vi "Actor Core Contents.vi"(8 "error in":errorcluster, 11 "Actor in":refnum<class "Actor.lvclass">) -> (0 "error out":errorcluster, 3 "Actor out":refnum<class "Actor.lvclass">)   [LabVIEW 2026, in "Lumberjack.lvlib" / "LogManager.lvclass"]
doc: "<p>(<strong>Filename</strong>: <span class=\"dnl\">Actor Framework.lvlib:Actor.lvclass:Actor Core.vi</span>)</p>\n<p>Receives messages to the actor, reacts to them, and initiates any error handling that may shut the actor down.</p>\n<p>Descendant classes may override this VI to append parallel tasks for the actor to complete while it handles messages. Overrides use the <a href=\"nihelplauncher://docs/csh?context=lvcore_glang_udclass\">Call Parent Class Method</a> node.</p>"
uses:
  LogManager.lvclass
  LogManager.lvclass/LogManager.ctl
  Appenders/Appender.lvclass/Appender.lvclass
  <vilib>/ActorFramework/Actor/Actor.lvclass
  C:/Program Files (x86)/National Instruments/LabVIEW 2026/vi.lib/ActorFramework/Actor/Actor.lvclass
  C:/Users/dallis/OneDrive - Velico Medical/Documents/Personal/LabVIEW Coding Projects/Lumberjack/src/Core/LogManager/LogManager.lvclass/LogManager.lvclass
  Layouts/CSVLayout.lvclass/CSVLayout.lvclass
  C:/Users/dallis/OneDrive - Velico Medical/Documents/Personal/LabVIEW Coding Projects/Lumberjack/src/Core/Layouts/Layout.lvclass/Layout.lvclass
  C:/Users/dallis/OneDrive - Velico Medical/Documents/Personal/LabVIEW Coding Projects/Lumberjack/src/Core/Layouts/CSVLayout.lvclass/CSVLayout.lvclass
  Appenders/FileAppender.lvclass/FileAppender.lvclass
  C:/Users/dallis/OneDrive - Velico Medical/Documents/Personal/LabVIEW Coding Projects/Lumberjack/src/Core/Appenders/Appender.lvclass/Appender.lvclass
  C:/Users/dallis/OneDrive - Velico Medical/Documents/Personal/LabVIEW Coding Projects/Lumberjack/src/Core/Appenders/FileAppender.lvclass/FileAppender.lvclass
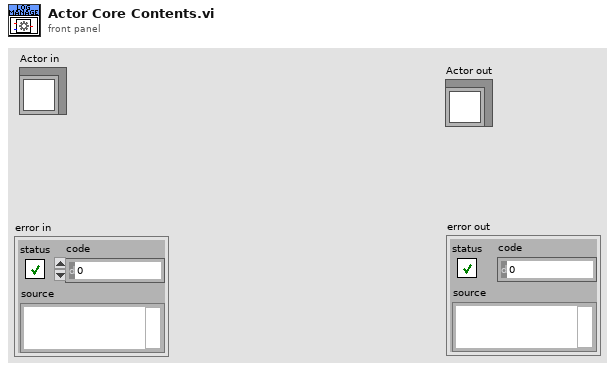
[diagram p1: front panel]
types:
  T1 = typedef "Lumberjack.lvlib/FileAppenderConfig.ctl" = cluster{"common":T2, "file":T7}
  T2 = typedef "Lumberjack.lvlib/AppenderConfig.ctl" = cluster{"id":string, "threshold":T3, "filter":T4, "queueBound":i32, "dropPolicy":T6, "useUTC":bool}
  T3 = typedef "Lumberjack.lvlib/Severity.ctl" = enum16{"OFF", "FATAL", "ERROR", "WARN", "INFO", "DEBUG", "TRACE", "ALL"}
  T4 = typedef "Lumberjack.lvlib/Filter.ctl" = cluster{"mode":T5, "levelMin":T3, "levelMax":T3, "tagPrefix":string}
  T5 = typedef "Lumberjack.lvlib/FilterMode.ctl" = enum16{"Mirror", "Routed"}
  T6 = typedef "Lumberjack.lvlib/DropPolicy.ctl" = enum16{"DropOldest", "DropNewest", "LevelAware"}
  T7 = typedef "Lumberjack.lvlib/FileConfig.ctl" = cluster{"rootFolder":path, "maxFileSize":i64, "maxFileCount":i32, "baseName":string, "extension":string, "delimiter":string, "calendarFolderTree":bool}
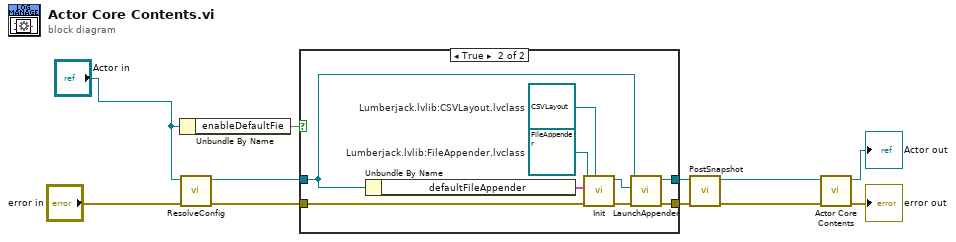
[diagram p0: block diagram]
diagram:
  n1 = Unbundle By Name("Actor in") -> ("enableDefaultFie"=w2)
  n2 = call "ResolveConfig.vi"("error in (no error)"="error in", "LogManager in"="Actor in") -> ("error out"=w7:errorcluster, "LogManager out"=w8:refnum<class "LogManager.lvclass">)  [unwired: 8 in]
  n3 = case shown="True" w2 {
    tunnel: w8 -> [w13 w15]
    tunnel: w7 -> [w12 w20]
    tunnel: [w13 w22] -> w6
    tunnel: [w12 w21] -> w5
    frame False {
    }
    frame True {
      w17 = refnum<class "CSVLayout.lvclass"> refnum  # Lumberjack.lvlib:CSVLayout.lvclass
      w18 = refnum<class "FileAppender.lvclass"> refnum  # Lumberjack.lvlib:FileAppender.lvclass
      n4 = Unbundle By Name(w15) -> ("defaultFileAppender"=w14:T1)
      n5 = call "Init.vi"("Lumberjack.lvlib:Layout.lvclass"=w17, "error in (no error)"=w20, "FileAppenderConfig"=w14, "FileAppender in"=w18) -> ("error out"=w19:errorcluster, "FileAppender out"=w16:refnum<class "FileAppender.lvclass">)  [unwired: 6 in]
      n6 = call "LaunchAppender.vi"("error in (no error)"=w19, "Lumberjack.lvlib:Appender.lvclass"=w16, "LogManager in"=w15) -> ("error out"=w21:errorcluster, "LogManager out"=w22:refnum<class "LogManager.lvclass">)  [unwired: 7 in]
    }
  }
  n7 = call "PostSnapshot.vi"("error in (no error)"=w5, "LogManager in"=w6) -> ("error out"=w3:errorcluster, "LogManager out"=w4:refnum<class "LogManager.lvclass">)  [unwired: 8 in]
  n8 = call-parent "Actor Core Contents.vi"("error in"=w3, "Actor in"=w4) -> ("error out"=→"error out":errorcluster, "Actor out"=→"Actor out":refnum<class "Actor.lvclass">)  [unwired: 8 in]
